vi "write_log_metadata.vi"(8 "error in (no error)":errorcluster, 10 "data":variant, 11 "hdf5_photon_record_log in":refnum<class "hdf5_photon_record_log.lvclass">) -> (0 "error out":errorcluster, 3 "hdf5_photon_record_log out":refnum<class "hdf5_photon_record_log.lvclass">)   [LabVIEW 2015, in "hdf5_photon_record_log.lvclass"]
uses:
  hdf5_photon_record_log.lvclass
  stream_metadata.ctl
  hydraharp_panel/hpanel_hydraharp_settings.ctl
  hydraharp_panel/hpanel_sync_settings.ctl
  hydraharp_panel/hpanel_sync_div.ctl
  hydraharp_panel/hpanel_channel_settings.ctl
  hdf5_photon_record_log.lvclass/hdf5_photon_record_log.ctl
  <vilib>/UPVI/lvhdf5/attribute.llb/Simple H5Awrite (Variant).vi
  <vilib>/UPVI/lvhdf5/attribute.llb/LVH5A Operation.ctl
  <vilib>/UPVI/lvhdf5/attribute.llb/Simple H5Awrite.xnode
  <vilib>/UPVI/lvhdf5/library.llb/HDF5 Ref.ctl
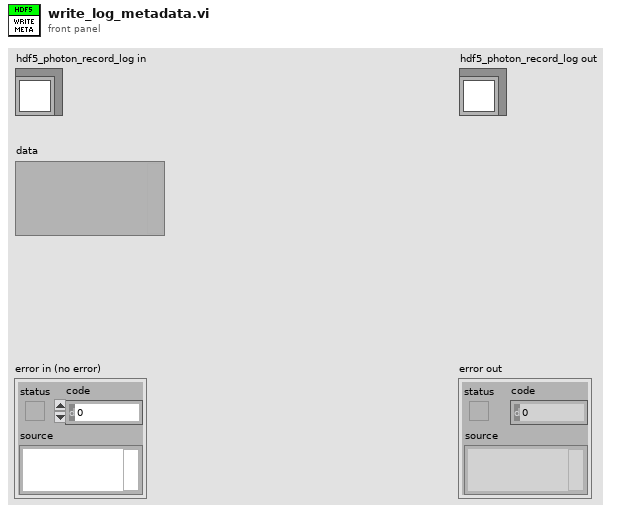
[diagram p1: front panel]
types:
  T1 = typedef "stream_metadata.ctl" = cluster{"Hydraharp Settings":T2, "resolution":dbl, "stream_notes":string}
  T2 = typedef "hpanel_hydraharp_settings.ctl" = cluster{"Sync Settings":T3, "CH 1":T5, "CH 2":T5, "CH 3":T5, "CH 4":T5, "binning":i32, "CH 5":T5, "CH 6":T5, "CH 7":T5, "CH 8":T5}
  T3 = typedef "hpanel_sync_settings.ctl" = cluster{"snc_count":i32, "snc_level":i32, "snc_ZeroX":i32, "snc_offs":i32, "sync_div":T4}
  T4 = typedef "hpanel_sync_div.ctl" = enum16{"1", "2", "4", "8"}
  T5 = typedef "hpanel_channel_settings.ctl" = cluster{"ch_counts":i32, "ch_level":i32, "ch_ZeroX":i32, "ch_offs":i32}
  T6 = typedef "HDF5 Ref.ctl" = refnum<k1>
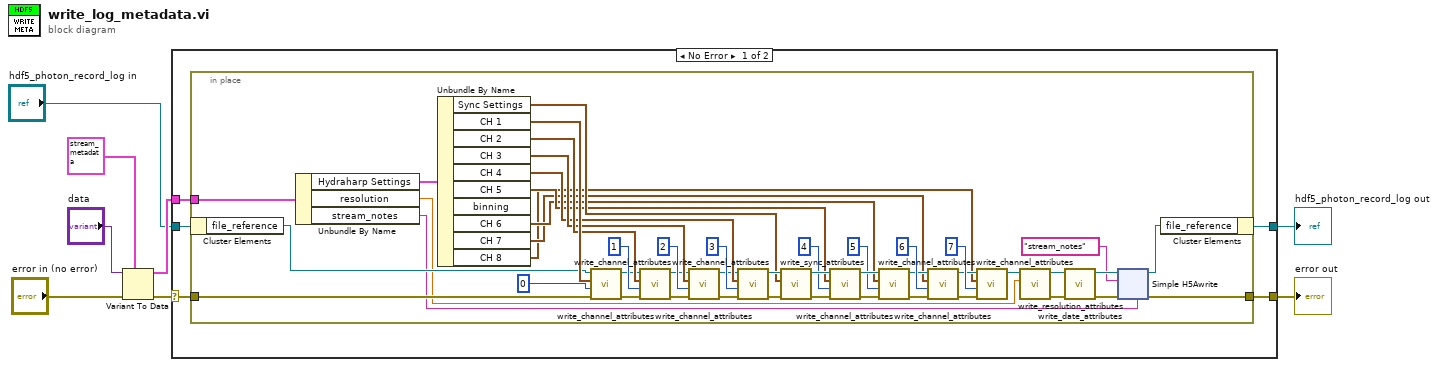
[diagram p0: block diagram]
diagram:
  n1 = Variant To Data(error in="error in (no error)", type=T1 {"Hydraharp Settings"={"Sync Settings"={"snc_count"=0, "snc_level"=0, "snc_ZeroX"=0, "snc_offs"=0, "sync_div"=enum."1"}, "CH 1"={"ch_counts"=0, "ch_level"=0, "ch_ZeroX"=0, "ch_offs"=0}, "CH 2"={"ch_counts"=0, "ch_level"=0, "ch_ZeroX"=0, "ch_offs"=0}, "CH 3"={"ch_counts"=0, "ch_level"=0, "ch_ZeroX"=0, "ch_offs"=0}, "CH 4"={"ch_counts"=0, "ch_level"=0, "ch_ZeroX"=0, "ch_offs"=0}, "binning"=0, "CH 5"={"ch_counts"=0, "ch_level"=0, "ch_ZeroX"=0, "ch_offs"=0}, "CH 6"={"ch_counts"=0, "ch_level"=0, "ch_ZeroX"=0, "ch_offs"=0}, "CH 7"={"ch_counts"=0, "ch_level"=0, "ch_ZeroX"=0, "ch_offs"=0}, "CH 8"={"ch_counts"=0, "ch_level"=0, "ch_ZeroX"=0, "ch_offs"=0}}, "resolution"=0.0, "stream_notes"="stream_notes"} ("output cluster"), Variant="data") -> (data=w6:T1, error out=w2:errorcluster)
  n2 = case shown="No Error" w2 {
    selector: w2 -> [w10 w76]
    tunnel: w6 -> [w11 _]
    tunnel: "hdf5_photon_record_log in" -> [w13 w77]
    tunnel: [w12 w77] -> w4
    tunnel: [w9 w76] -> w1
    frame No Error {
      n3 = in-place {
        in-place-border: w11 -> [w60]
        in-place-border: w10 -> [w40]
        in-place-border: [w16] -> w9
        n4 = in-place-cluster #1(w13) -> ("file_reference"=w50:T6)
        n5 = Unbundle By Name(w60) -> ("Hydraharp Settings"=w59:T2, "resolution"=w39:dbl, "stream_notes"=w14:string)
        n6 = Unbundle By Name(w59) -> ("Sync Settings"=w45:T3, "CH 1"=w58:T5, "CH 2"=w57:T5, "CH 3"=w56:T5, "CH 4"=w55:T5, "CH 5"=w23:T5, "CH 6"=w22:T5, "CH 7"=w21:T5, "CH 8"=w20:T5)  [unwired: 1 out]
        n7 = call "write_channel_attributes.vi"("error in (no error)"=w40, "ch_number"=0, "Hydraharp Settings.CH 0"=w58, "HDF5 Ref"=w50) -> ("error out"=w41:errorcluster, "HDF5 Ref out"=w49:T6)  [unwired: 6 in]
        n8 = call "write_channel_attributes.vi"("error in (no error)"=w41, "ch_number"=1, "Hydraharp Settings.CH 0"=w57, "HDF5 Ref"=w49) -> ("error out"=w42:errorcluster, "HDF5 Ref out"=w48:T6)  [unwired: 6 in]
        n9 = call "write_channel_attributes.vi"("error in (no error)"=w42, "ch_number"=2, "Hydraharp Settings.CH 0"=w56, "HDF5 Ref"=w48) -> ("error out"=w43:errorcluster, "HDF5 Ref out"=w47:T6)  [unwired: 6 in]
        n10 = call "write_channel_attributes.vi"("error in (no error)"=w43, "ch_number"=3, "Hydraharp Settings.CH 0"=w55, "HDF5 Ref"=w47) -> ("error out"=w44:errorcluster, "HDF5 Ref out"=w46:T6)  [unwired: 6 in]
        n11 = call "write_sync_attributes.vi"("error in (no error)"=w44, "Hydraharp Settings.Sync Settings"=w45, "HDF5 Ref"=w46) -> ("error out"=w28:errorcluster, "HDF5 Ref out"=w27:T6)  [unwired: 7 in]
        n12 = call "write_channel_attributes.vi"("error in (no error)"=w28, "ch_number"=4, "Hydraharp Settings.CH 0"=w23, "HDF5 Ref"=w27) -> ("error out"=w29:errorcluster, "HDF5 Ref out"=w34:T6)  [unwired: 6 in]
        n13 = call "write_channel_attributes.vi"("error in (no error)"=w29, "ch_number"=5, "Hydraharp Settings.CH 0"=w22, "HDF5 Ref"=w34) -> ("error out"=w30:errorcluster, "HDF5 Ref out"=w33:T6)  [unwired: 6 in]
        n14 = call "write_channel_attributes.vi"("error in (no error)"=w30, "ch_number"=6, "Hydraharp Settings.CH 0"=w21, "HDF5 Ref"=w33) -> ("error out"=w31:errorcluster, "HDF5 Ref out"=w32:T6)  [unwired: 6 in]
        n15 = call "write_channel_attributes.vi"("error in (no error)"=w31, "ch_number"=7, "Hydraharp Settings.CH 0"=w20, "HDF5 Ref"=w32) -> ("HDF5 Ref out"=w26:T6)  [unwired: 6 in, 1 out]
        n16 = call "write_resolution_attributes.vi"("resolution"=w39, "HDF5 Ref"=w26) -> ("error out"=w37:errorcluster, "HDF5 Ref out"=w38:T6)  [unwired: 8 in]
        n17 = call "write_date_attributes.vi"("error in (no error)"=w37, "HDF5 Ref"=w38) -> ("error out"=w19:errorcluster, "HDF5 Ref out"=w18:T6)  [unwired: 8 in]
        n18 = xnode "Simple H5Awrite"("HDF5 Ref"=w18, "Name"="stream_notes", "error in (no error)"=w19, "Value"=w14) -> ("HDF5 Ref out"=w17:T6, "error out"=w16:errorcluster)  [unwired: 1 in]
        n19 = in-place-cluster #1("file_reference"=w17) -> (w12:refnum<class "hdf5_photon_record_log.lvclass">)
      }
    }
    frame Error {
    }
  }
  "error out" <- w1
  "hdf5_photon_record_log out" <- w4
